vi "randomMove.vi"(6 "nMoves":i32, 7 "availables":i32[][](array[numeric])=[[0, 0, 0, 0, 0, 0, 0, 0], [0, 0, 0, 0, 0, 0, 0, 0], [0, 0, 0, 0, 0, 0, 0, 0], [0, 0, 0, 0, 0, 0, 0, 0], [0, 0, 0, 0, 0, 0, 0, 0], [0, 0, 0, 0, 0, 0, 0, 0], [0, 0, 0, 0, 0, 0, 0, 0], [0, 0, 0, 0, 0, 0, 0, 0], [0, 0, 0, 0, 0, 0, 0, 0]], 8 "pos":i32[][](array[numeric])=[[0, 0, 0, 0, 0, 0, 0, 0], [0, 0, 0, 0, 0, 0, 0, 0], [0, 0, 0, 0, 0, 0, 0, 0], [0, 0, 0, 0, 0, 0, 0, 0], [0, 0, 0, 0, 0, 0, 0, 0], [0, 0, 0, 0, 0, 0, 0, 0], [0, 0, 0, 0, 0, 0, 0, 0], [0, 0, 0, 0, 0, 0, 0, 0], [0, 0, 0, 0, 0, 0, 0, 0]], 9 "exist":i32[][](array[numeric])=[[0, 0, 0, 0, 0, 0, 0, 0], [0, 0, 0, 0, 0, 0, 0, 0], [0, 0, 0, 0, 0, 0, 0, 0], [0, 0, 0, 0, 0, 0, 0, 0], [0, 0, 0, 0, 0, 0, 0, 0], [0, 0, 0, 0, 0, 0, 0, 0], [0, 0, 0, 0, 0, 0, 0, 0], [0, 0, 0, 0, 0, 0, 0, 0], [0, 0, 0, 0, 0, 0, 0, 0]], 10 "mY":i32, 11 "mX":i32) -> (0 "posNew":i32[][](array[numeric]), 1 "existNew":i32[][](array[numeric]), 2 "mYNew":i32, 3 "mXNew":i32, 4 "randomMove":bool=TRUE, 5 "availablesNew":i32[][](array[numeric]))   [LabVIEW 2022 SP3, in "subvis.lvlib"]
uses:
  subvis.lvlib
panel:
  out "break":bool=TRUE
  out "ith":u32
  out "k":u32
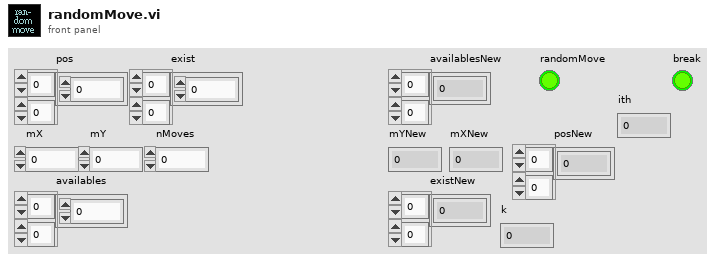
[diagram p1: front panel]
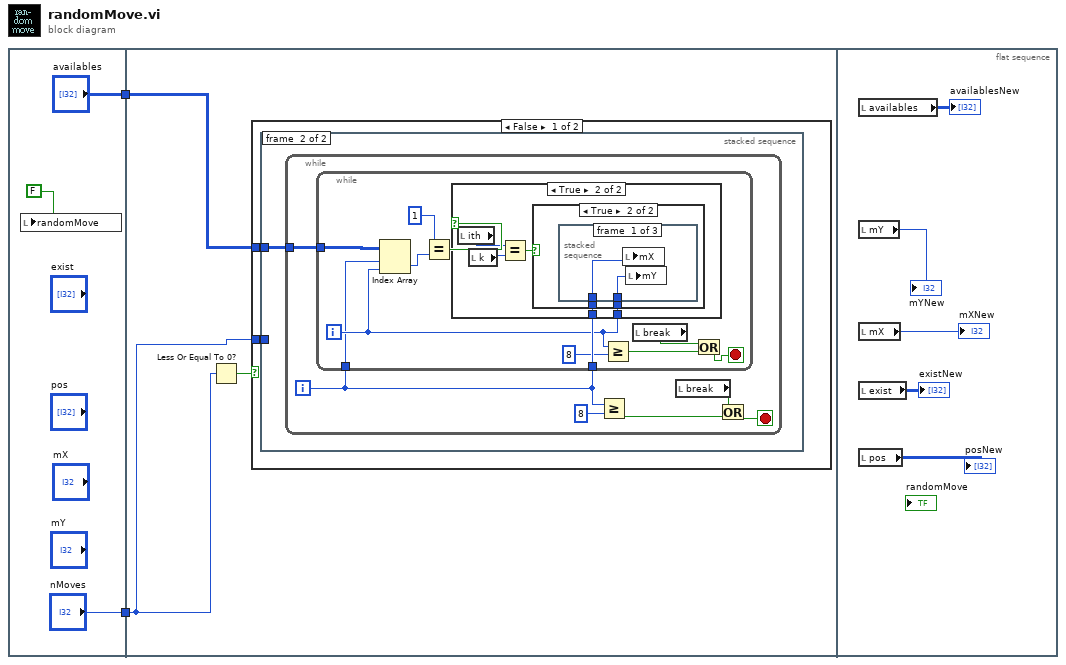
[diagram p0: block diagram]
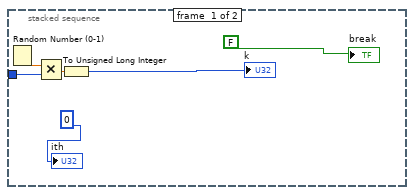
[diagram p2: hidden frame]
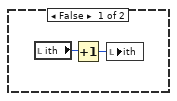
[diagram p4: hidden frame]
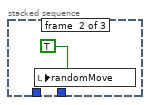
[diagram p5: hidden frame]
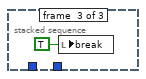
[diagram p6: hidden frame]
diagram:
  n1 = flat-sequence {
    tunnel: ["nMoves"] -> w2
    tunnel: ["availables"] -> w1
    tunnel: w2 -> [w7]
    tunnel: w1 -> [w6]
    frame #0 {
      n2 = local write "randomMove"(FALSE ("randomMove")) -> ()
    }
    frame #1 {
      n3 = Less Or Equal To 0?(x=w7) -> (x <= 0?=w8:bool)
      n4 = case shown="False" w8 {
        tunnel: w7 -> [w10 _]
        tunnel: w6 -> [w9 _]
        frame False {
          n5 = stacked-sequence {
            tunnel: w10 -> [w13 _]
            tunnel: w9 -> [_ w17]
            frame #0 {
              n6 = Random Number (0-1)() -> (number: 0 to 1=w14:dbl)
              n7 = Multiply(x=w14, y=w13) -> (x*y=w15:dbl)
              n8 = To Unsigned Long Integer(number=w15) -> (unsigned 32bit integer=→"k":u32)
              "ith" <- u32 0 ("ith")
              "break" <- FALSE
            }
            frame #1 {
              n9 = while {
                tunnel: w17 -> [w19]
                i -> [w18]
                stop <- w21 stop-if-true
                n10 = while {
                  tunnel: w18 -> [w34]
                  tunnel: w19 -> [w29]
                  tunnel: w18 -> [w27]
                  i -> [w28]
                  stop <- w32 stop-if-true
                  n11 = Index Array(array=w29, index (row)=w27, index (col)=w28) -> (element=w26:i32)
                  n12 = Equal?(x=1, y=w26) -> (x = y?=w24:bool)
                  n13 = case shown="True" w24 {
                    tunnel: w28 -> [_ w39]
                    tunnel: w34 -> [_ w38]
                    frame False {
                    }
                    frame True {
                      n14 = local read "ith"() -> (w37:u32)
                      n15 = local read "k"() -> (w36:u32)
                      n16 = Equal?(x=w37, y=w36) -> (x = y?=w35:bool)
                      n17 = case shown="True" w35 {
                        tunnel: w39 -> [_ w43]
                        tunnel: w38 -> [_ w42]
                        frame False {
                          n18 = local read "ith"() -> (w41:u32)
                          n19 = Increment(x=w41) -> (x+1=w40:u32)
                          n20 = local write "ith"(w40) -> ()
                        }
                        frame True {
                          n21 = stacked-sequence {
                            tunnel: w43 -> [w45 _ _]
                            tunnel: w42 -> [w44 _ _]
                            frame #0 {
                              n22 = local write "mX"(w44) -> ()
                              n23 = local write "mY"(w45) -> ()
                            }
                            frame #1 {
                              n24 = local write "randomMove"(TRUE ("randomMove")) -> ()
                            }
                            frame #2 {
                              n25 = local write "break"(TRUE ("break")) -> ()
                            }
                          }
                        }
                      }
                    }
                  }
                  n26 = Greater Or Equal?(x=w28, y=8) -> (x >= y?=w30:bool)
                  n27 = local read "break"() -> (w31:bool)
                  n28 = Or(x=w31, y=w30) -> (x .or. y?=w32:bool)
                }
                n29 = Greater Or Equal?(x=w18, y=8) -> (x >= y?=w20:bool)
                n30 = local read "break"() -> (w22:bool)
                n31 = Or(x=w22, y=w20) -> (x .or. y?=w21:bool)
              }
            }
          }
        }
        frame True {
        }
      }
    }
    frame #2 {
      n32 = local read "availables"() -> (→"availablesNew":i32[][])
      n33 = local read "mY"() -> (→"mYNew":i32)
      n34 = local read "mX"() -> (→"mXNew":i32)
      n35 = local read "exist"() -> (→"existNew":i32[][])
      n36 = local read "pos"() -> (→"posNew":i32[][])
    }
  }
